vi "Add Struture Project Items.vi"(8 "error in (no error)":errorcluster, 10 "Folder Location Ref":refnum<vi>, 11 "Block Diagram in":refnum<class "VI.lvclass">) -> (0 "error out":errorcluster, 3 "Block Diagram out":refnum<class "VI.lvclass">)   [LabVIEW 2015, in "VI.lvclass"]
uses:
  VI.lvclass
  VI.lvclass/VI.ctl
  Structures/Structures.lvclass
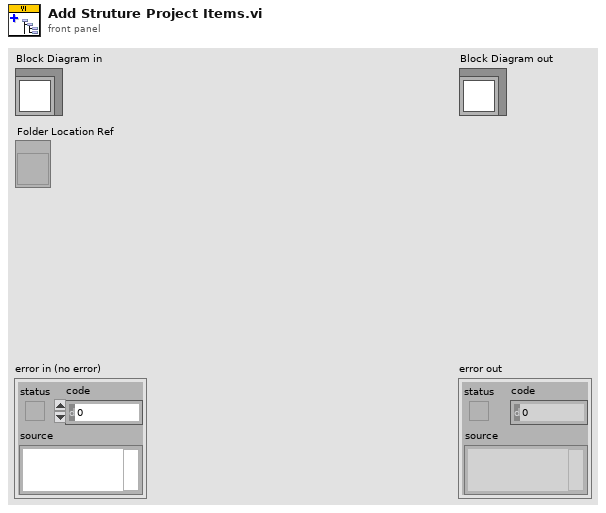
[diagram p1: front panel]
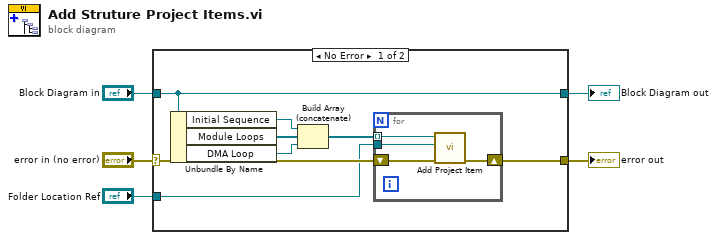
[diagram p0: block diagram]
diagram:
  n1 = case shown="No Error" "error in (no error)" {
    selector: "error in (no error)" -> [w11 w19]
    tunnel: [w10 w19] -> w4
    tunnel: [w13 w18] -> w2
    tunnel: "Block Diagram in" -> [w13 w18]
    tunnel: "Folder Location Ref" -> [w9 _]
    frame No Error {
      n2 = Unbundle By Name(w13) -> ("Initial Sequence"=w6:refnum<class "Main Sequence.lvclass">, "Module Loops"=w12:refnum<class "Module Loop.lvclass">[], "DMA Loop"=w7:refnum<class "DMA Loop.lvclass">)
      n3 = Build Array (concatenate)(w6, w12, w7) -> (w8:refnum<class "Structures.lvclass">[])
      n4 = for {
        tunnel: w8 -> [w17] mode=indexing
        shift-right: [w15] -> w10
        shift-left: w11 -> [w16]
        tunnel: w9 -> [w14]
        n5 = call-dynamic "Add Project Item.vi"("error in (no error)"=w16, "Folder Location Ref"=w14, "Structures in"=w17) -> ("error out"=w15:errorcluster)  [unwired: 7 in, 1 out]
      }
    }
    frame Error {
    }
  }
  "error out" <- w4
  "Block Diagram out" <- w2
